vi "FT3 Main.vi"() -> ()   [LabVIEW 2014]
panel:
  in  "Numeric 2":dbl
  in  "Numeric":dbl
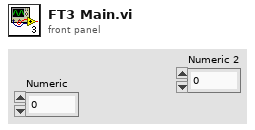
[diagram p1: front panel]
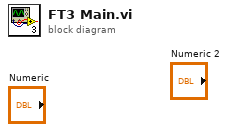
[diagram p0: block diagram]
diagram:
